vi "GetNextScheduledSlot.vi"(1 "Time Stamp":timestamp, 2 "Array":T1(array[cluster]) {"End" format="%<%.3X>T"; "Start" format="%<%.3X>T"}) -> (0 "Numeric":dbl)   [LabVIEW 2017]
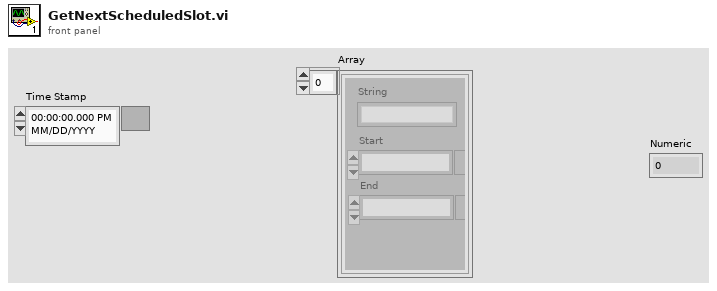
[diagram p1: front panel]
types:
  T1 = cluster{"String":string, "Start":timestamp, "End":timestamp}[]
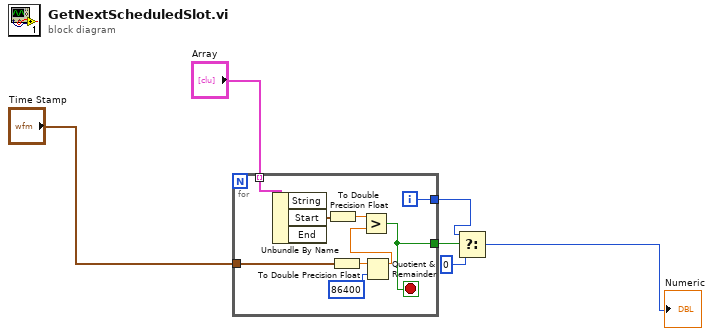
[diagram p0: block diagram]
diagram:
  n1 = for {
    tunnel: "Array" -> [w15] mode=indexing
    tunnel: [w9] -> w4
    tunnel: [w8] -> w6
    tunnel: "Time Stamp" -> [w7]
    i -> [w8]
    stop <- w9 stop-if-true
    n2 = Unbundle By Name(w15) -> ("Start"=w12:timestamp)  [unwired: 2 out]
    n3 = To Double Precision Float(number=w12) -> (double precision float=w11:dbl)
    n4 = To Double Precision Float(number=w7) -> (double precision float=w14:dbl)
    n5 = Quotient & Remainder(x=w14, y=86400) -> (x-y*floor(x/y)=w10:dbl)  [unwired: 1 out]
    n6 = Greater?(x=w11, y=w10) -> (0:w9:bool)
  }
  n7 = Select(t=w6, s=w4, f=0) -> (s? t:f=→"Numeric":i32)
